vi "Set Shed Sequence.vi"(8 "error in (no error)":errorcluster, 11 "SCADA in":refnum<class "SCADA.lvclass">) -> (0 "error out":errorcluster, 3 "SCADA out":refnum<class "SCADA.lvclass">)   [LabVIEW 2015, in "SCADA Core.lvlib" / "SCADA.lvclass"]
uses:
  SCADA.lvclass
  <vilib>/ActorFramework/Actor/Actor.lvclass/Actor.ctl
  SCADA.lvclass/SCADA.ctl
  SCADA Abstract Messages/Set Shed Sequence Status Msg/Set Shed Sequence Status.ctl
  <vilib>/NI/Tools/Keyed Array/Map String.vi
  <vilib>/NI/Tools/String/Get Case Matching.vi
  <vilib>/NI/Tools/Keyed Array/Tools_KeyedArray.lvlib
  <vilib>/ActorFramework/Actor/Actor.lvclass
  SCADA Abstract Messages/Set Shed Sequence Status Msg/Set Shed Sequence Status Msg.lvclass
panel:
  in  "Sequence":string
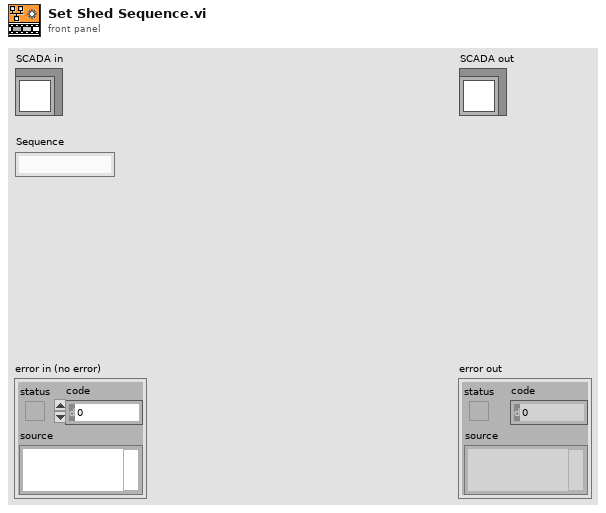
[diagram p1: front panel]
types:
  T1 = typedef "SCADA Core.lvlib/Set Shed Sequence Status Msg.lvclass/Set Shed Sequence Status.ctl" = enum16{"Success", "Failure"}
  T2 = typedef "Tools_KeyedArray.lvlib/KeyedArray.ctl" = cluster{"keys":string[], "values":string[]}
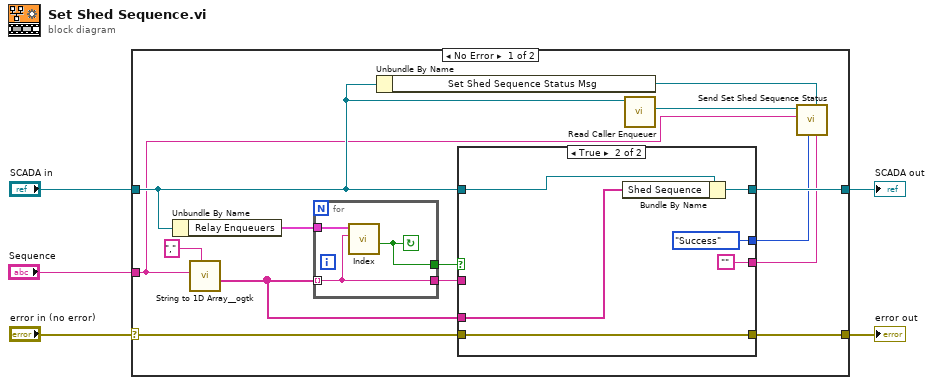
[diagram p0: block diagram]
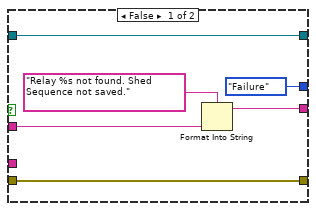
[diagram p2: hidden frame]
diagram:
  n1 = case shown="No Error" "error in (no error)" {
    selector: "error in (no error)" -> [w16 w36]
    tunnel: [w14 w36] -> w4
    tunnel: [w13 w35] -> w2
    tunnel: "SCADA in" -> [w12 w35]
    tunnel: "Sequence" -> [w9 _]
    frame No Error {
      n2 = Unbundle By Name(w12) -> ("Relay Enqueuers"=w18:T2)
      n3 = call <userlib>:"String to 1D Array__ogtk.vi"("delimiter (Tab)"=",", "string"=w9) -> ("Array of Strings"=w15:string[])  [unwired: 9 in]
      n4 = for {
        tunnel: w18 -> [w34]
        tunnel: w15 -> [w32] mode=indexing
        tunnel: [w33] -> w17
        tunnel: [w32] -> w8
        stop <- w33 continue-if-true
        n5 = call <vilib>:"Index.vi"("key"=w32, "array in"=w34) -> ("valid key"=w33:bool)  [unwired: 3 in, 2 out]
      }
      n6 = Unbundle By Name(w12) -> ("Set Shed Sequence Status Msg"=w10:refnum<class "Set Shed Sequence Status Msg.lvclass">)
      n7 = case shown="True" w17 {
        tunnel: w16 -> [w24 w31]
        tunnel: w15 -> [_ w29]
        tunnel: w12 -> [w25 w30]
        tunnel: [w24 w31] -> w14
        tunnel: [w25 w28] -> w13
        tunnel: w8 -> [w22 _]
        tunnel: [w21 ""] -> w7
        tunnel: [Set_Shed_Sequence_Status."Failure" ("Status") Set_Shed_Sequence_Status."Success" ("Status")] -> w6
        frame False {
          n8 = Format Into String(format string="Relay %s not found. Shed Sequence not saved.", w22) -> (resulting string=w21:string)  [unwired: 2 in, 1 out]
        }
        frame True {
          n9 = Bundle By Name(cluster=w30, "Shed Sequence"=w29) -> (w28:refnum<class "SCADA.lvclass">)
        }
      }
      n10 = call <vilib>:"Read Caller Enqueuer.vi"("Actor"=w12) -> ("Caller Enqueuer"=w11:refnum<class "Message Enqueuer.lvclass">)  [unwired: 10 in]
      n11 = call "Send Set Shed Sequence Status.vi"("error"=w7, "Set Shed Sequence Status Msg"=w10, "Status"=w6, "Sequence"=w9, "Message Enqueuer in"=w11) -> ()  [unwired: 5 in, 2 out]
    }
    frame Error {
    }
  }
  "error out" <- w4
  "SCADA out" <- w2
